vi "Test Stop.vi"(11 "Error in":errorcluster) -> (15 "Error out":errorcluster)   [LabVIEW 2020, in "CelsiusToFarenheitTests.lvlib"]
doc: "This VI is to validate the stop button"
uses:
  CelsiusToFarenheitTests.lvlib
  <vilib>/SLL Drona/APIs/Assert/AssertVI/AssertVIExecRunning.vi
  <vilib>/SLL Drona/APIs/Stimulus/ControlValue/SetValueAuto.vi
  <vilib>/SLL Drona/APIs/Assert/AssertVI/AssertVIExecIdle.vi
  <vilib>/SLL Drona/APIs/Stimulus/VI/CloseVI.vi
  <vilib>/Utility/error.llb/Error Cluster From Error Code.vi
  <vilib>/ErrorRing/Error Ring.xnode
  <vilib>/SLL Drona/Drona.lvlib
  <vilib>/addons/_JKI Toolkits/Caraya/classes/Test/Test.lvclass
  <vilib>/Wiresmith Technology/G CLI/CLI Class/CLI.lvclass
  <vilib>/SLL Drona/APIs/Assert/AssertVI/AssertVI.lvlib
  <vilib>/SLL Drona/APIs/Stimulus/VI/VI.lvlib
  <vilib>/SLL Drona/APIs/Stimulus/ControlValue/ControlValue.lvlib
panel:
  # "STOP BUTTON TEST"
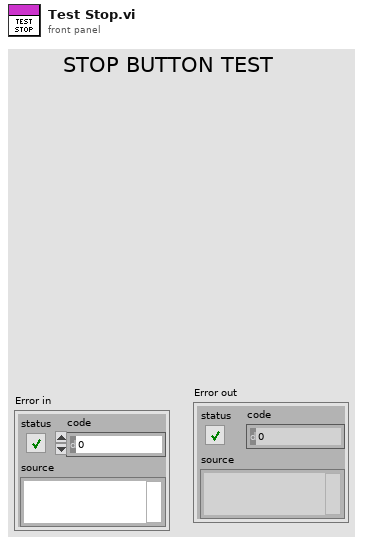
[diagram p1: front panel]
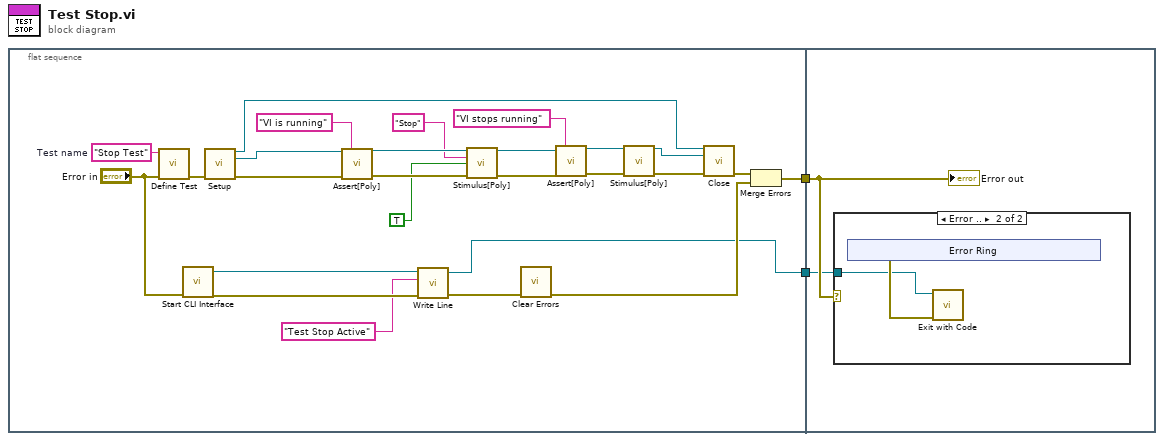
[diagram p0: block diagram]
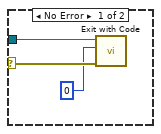
[diagram p2: hidden frame]
diagram:
  n1 = flat-sequence {
    tunnel: [w6] -> w2
    tunnel: [w3] -> w1
    tunnel: w2 -> [w30]
    tunnel: w1 -> [w29]
    frame #0 {
      w27 = "Stop Test"  # Test name
      n2 = call <vilib>:"Define Test.vi"("error in (no error)"="Error in", "Label (VI Title)"=w27) -> ("error out"=w28:errorcluster)  [unwired: 9 in]
      n3 = call <vilib>:"Start CLI Interface.vi"("error in (no error)"="Error in") -> ("error out"=w10:errorcluster, "CLI out"=w9:refnum<class "CLI.lvclass">)  [unwired: 7 in, 2 out]
      n4 = call <vilib>:"Setup.vi"("error in"=w28) -> ("Application Ref"=w26:refnum<vi>, "VI Reference Out"=w23:refnum<vi>, "error out"=w13:errorcluster)  [unwired: 12 in]
      n5 = call-poly <vilib>:"Assert[Poly].vi"("VI Reference In"=w23, "Test Label"="VI is running", "Error In"=w13) -> ("VI Reference Out"=w21:refnum<vi>, "Error Out"=w22:errorcluster)  [unwired: 11 in]
      n6 = call <vilib>:"Write Line.vi"("error in (no error)"=w10, "Text to Write"="Test Stop Active", "CLI in"=w9) -> ("error out"=w5:errorcluster, "CLI out"=w3:refnum<class "CLI.lvclass">)  [unwired: 7 in]
      n7 = call-poly <vilib>:"Stimulus[Poly].vi"("VI Reference In"=w21, "Control Path"="Stop", "Value (Signaling)"=TRUE, "error in"=w22) -> ("VI Reference Out"=w17:refnum<vi>, "error out"=w18:errorcluster)  [unwired: 10 in]
      n8 = call <vilib>:"Clear Errors.vi"("error in (no error)"=w5) -> ("error out"=w4:errorcluster)  [unwired: 5 in, 1 out]
      n9 = call-poly <vilib>:"Assert[Poly].vi"("VI Reference In"=w17, "Test Label"="VI stops running", "Error In"=w18) -> ("VI Reference Out"=w14:refnum<vi>, "Error Out"=w15:errorcluster)  [unwired: 11 in]
      n10 = call-poly <vilib>:"Stimulus[Poly].vi"("VI Reference In"=w14, "error in"=w15) -> ("VI Reference Out"=w25:refnum<vi>, "error out"=w12:errorcluster)  [unwired: 12 in]
      n11 = call <vilib>:"Close.vi"("Application Ref"=w26, "VI Reference"=w25, "error in"=w12) -> ("error out"=w7:errorcluster)  [unwired: 12 in]
      n12 = Merge Errors(w7, w4) -> (w6:errorcluster)
    }
    frame #1 {
      n13 = case shown="Error .." w30 {
        selector: w30 -> [w33 _]
        tunnel: w29 -> [w32 w34]
        frame No Error {
          n14 = call <vilib>:"Exit with Code.vi"("error in (no error)"=w33, "Exit Code (0)"=0, "CLI in"=w32) -> ()  [unwired: 8 in, 1 out]
        }
        frame Error {
          n15 = xnode "Error Ring"() -> ("error out"=w35:errorcluster)
          n16 = call <vilib>:"Exit with Code.vi"("error in (no error)"=w35, "CLI in"=w34) -> ()  [unwired: 9 in, 1 out]
        }
      }
      "Error out" <- w30
    }
  }
